vi "wavtest.vi"() -> ()   [LabVIEW 2016]
uses:
  <vilib>/Instr/_visa.llb/VISA Configure Serial Port (Instr).vi
  <vilib>/measure/maspectr.llb/FFT Spectrum (Mag-Phase) for 1 Chan.vi
  <vilib>/Waveform/WDTOps.llb/WDT Append Waveforms DBL.vi
  <vilib>/measure/NI_MAPro.lvlib
panel:
  out "VISA name":refnum<visa-resource-name>
  out "JSON string 2":string
  out "JSON string":string
  out "Para Cubo 2":dbl[][](array[numeric])
  out "# found 2":i32
  out "Janela 2":waveform(dbl)(graph)
  out "Amp 2":cluster{"f0":dbl, "df":dbl, "magnitude":dbl[]}(graph) caption="Amp"
  out "Raw Wave 2":waveform(dbl)(graph)
  in  "Record Button":bool caption="Gravar"
  in  "Close":bool
  out "Para Cubo":dbl[][](array[numeric])
  out "# found":i32
  in  "Tempo de Amostra do Som":dbl=0.01 min=0.05 max=1.0 step=0.01 format="%#_13g"
  out "Max iter":i32
  out "Ele/0,1s":dbl
  out "dt":dbl
  out "Duração Total":dbl
  out "size(s)":i32
  out "error out":errorcluster
  out "Janela":waveform(dbl)(graph)
  out "Amp":cluster{"f0":dbl, "df":dbl, "magnitude":dbl[]}(graph)
  in  "Play Button":bool
  out "Raw Wave":waveform(dbl)(graph)
  in  "Path to wav song":path caption="Escolher Arquivo"
  out "Menu 1":u32(colorbox)
  out "Ajustes":u32(colorbox)
  out "Back":u32(colorbox)
  # "Ajustes"
  # "PSI3214 -\nLaboratório de\nInstrumentação\nElétrica                 2016"
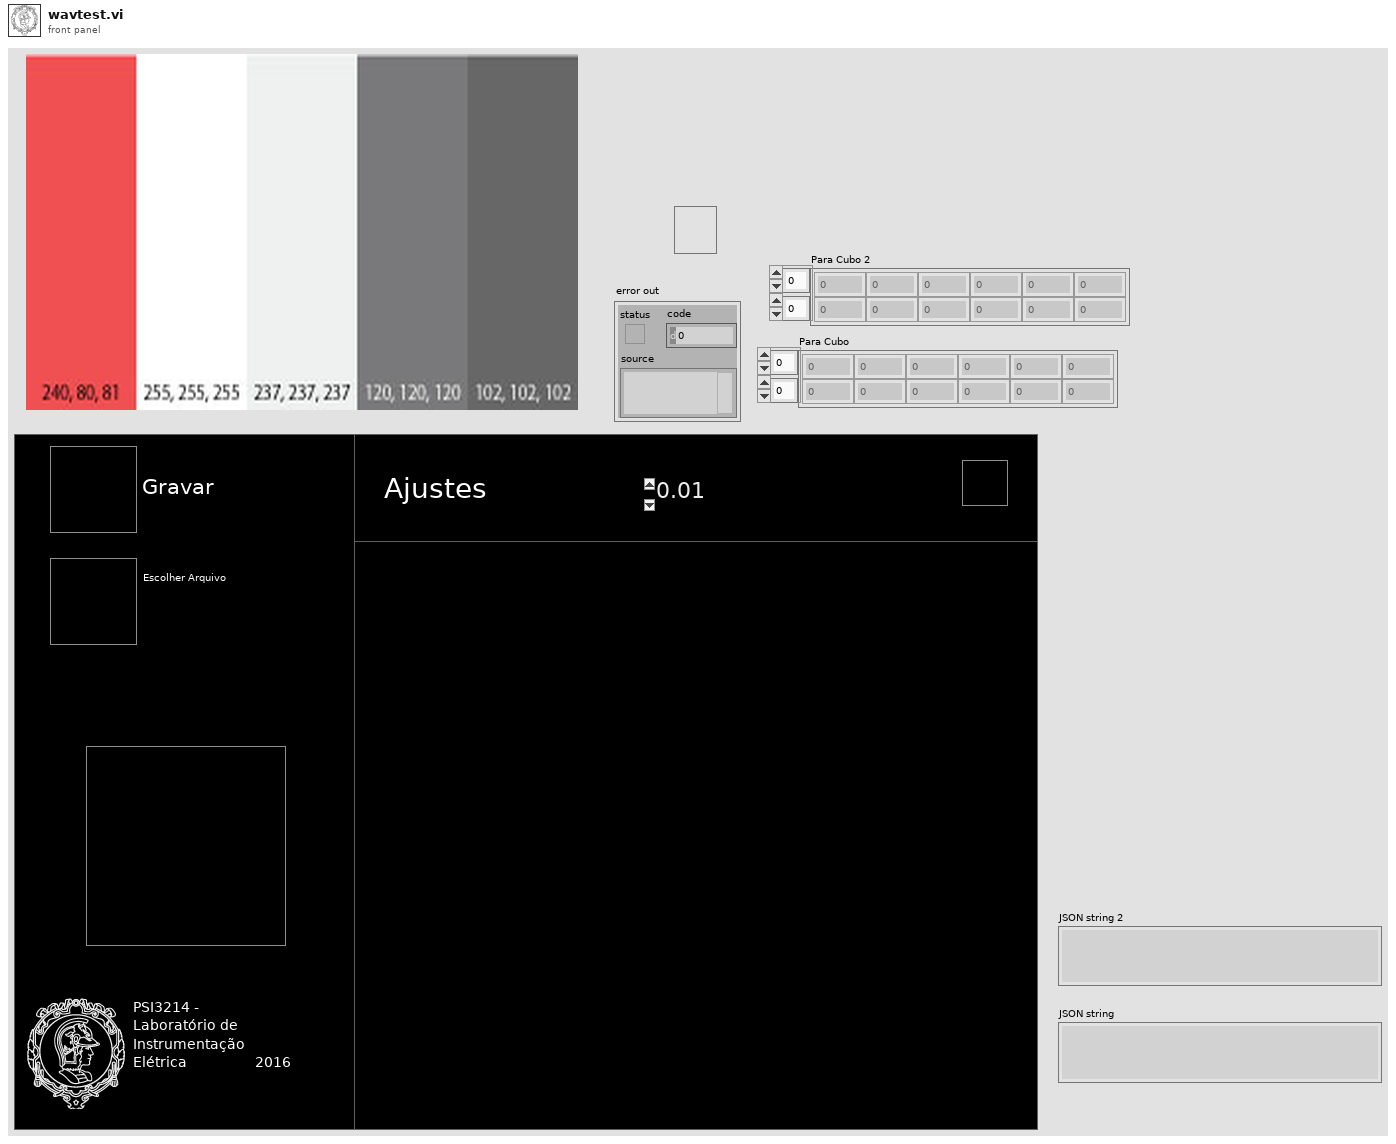
[diagram p1: front panel]
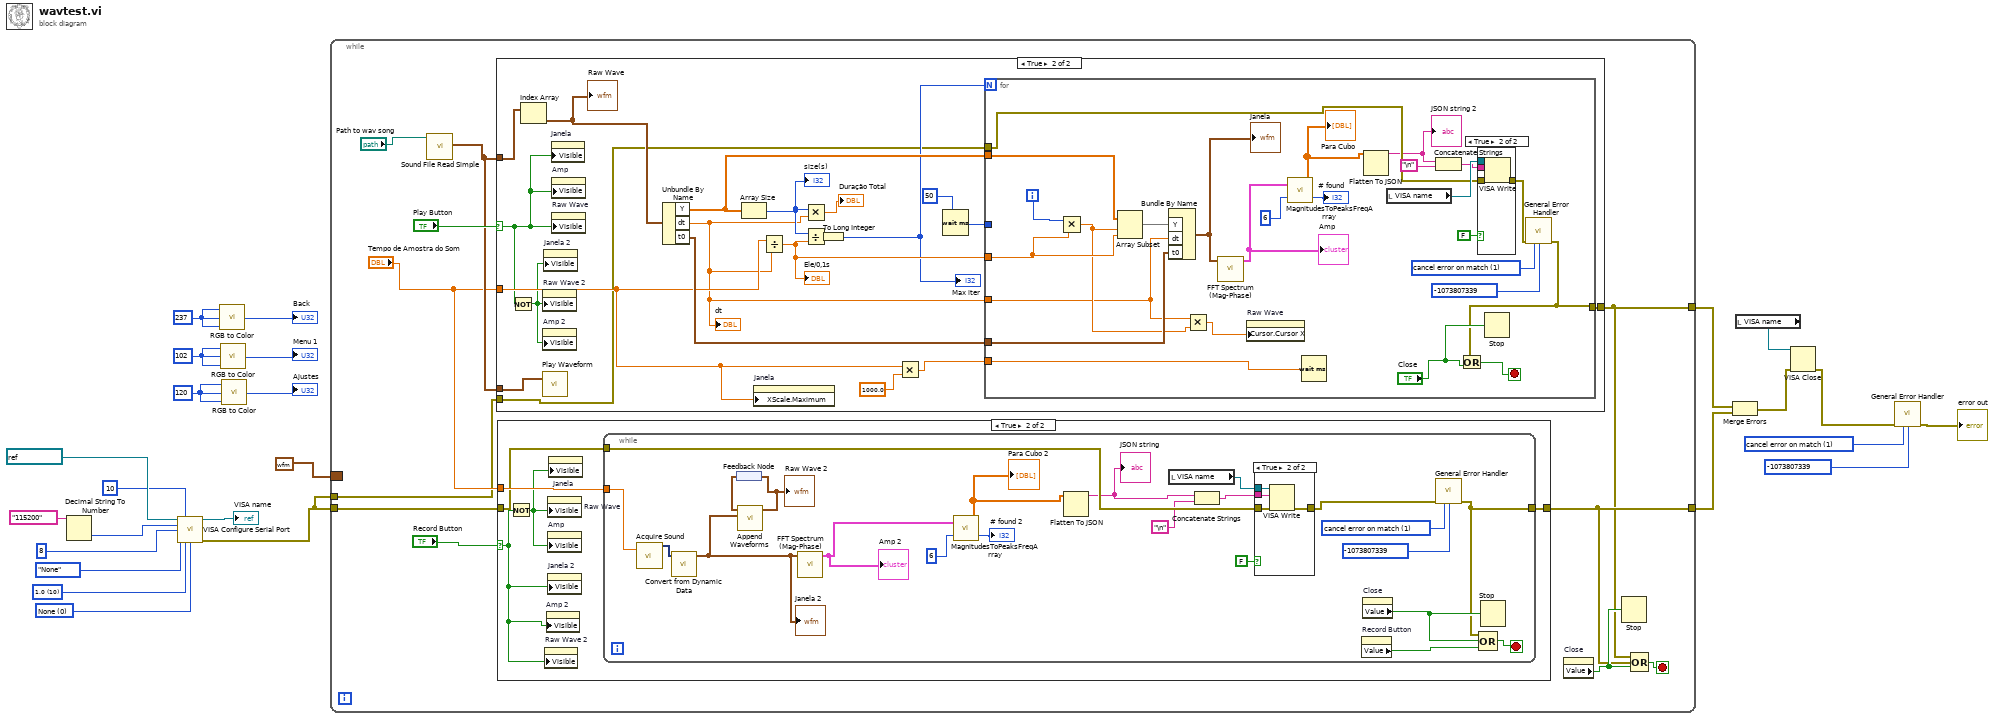
[diagram p0: block diagram]
diagram:
  w2 = 1 items=["no exception", "cancel error on match", "set error on match"] ("[exception action] (none:0)")
  w14 = u16 0 items=["None", "XON/XOFF", "RTS/CTS", "XON/XOFF & RTS/CTS", "DTR/DSR", "XON/XOFF & DTR/DSR"] ("flow control (0:none)")
  w15 = u16 10 items=["1.0"=10, "1.5"=15, "2.0"=20] ("stop bits (10: 1 bit)")
  w19 = u8 120 ("G")
  w20 = u8 102 ("G")
  w21 = u8 237 ("G")
  n1 = Decimal String To Number(string="115200" ("Baud Rate")) -> (number=w12:i32)  [unwired: 2 in, 1 out]
  n2 = call-poly "VISA Configure Serial Port"("VISA resource name"=refnum<visa-resource-name> "COM18" ("COM Port"), "timeout (10sec)"=u32 10, "baud rate (9600)"=w12, "data bits (8)"=u16 8, "parity (0:none)"=enum16{"None", "Odd", "Even", "Mark", "Space"}."None", "stop bits (10: 1 bit)"=w15, "flow control (0:none)"=w14) -> ("VISA resource name out"=→"VISA name":refnum<visa-resource-name>, "error out"=w4:errorcluster)  [unwired: 7 in]
  n3 = call <vilib>:"RGB to Color.vi"("B"=w21, "G"=w21, "R"=w21) -> ("Color"=→"Back":u32)
  n4 = call <vilib>:"RGB to Color.vi"("B"=w20, "G"=w20, "R"=w20) -> ("Color"=→"Menu 1":u32)
  n5 = call <vilib>:"RGB to Color.vi"("B"=w19, "G"=w19, "R"=w19) -> ("Color"=→"Ajustes":u32)
  n6 = while {
    border: waveform(dbl) {"t0"=timestamp(0 s since 1904-01-01), "dt"=1.0, "Y"=[]} ("waveform out") -> [_]
    tunnel: [w26] -> w7
    tunnel: [w27] -> w6
    tunnel: w4 -> [w31]
    tunnel: w4 -> [w30]
    stop <- w28 stop-if-true
    n7 = call <vilib>:"Sound File Read Simple.vi"("path"="Path to wav song") -> ("data"=w35:waveform(dbl)[])  [unwired: 7 in, 3 out]
    n8 = case shown="True" "Play Button" {
      selector: "Play Button" -> [_ w73]
      tunnel: w35 -> [_ w90]
      tunnel: "Tempo de Amostra do Som" -> [_ w79]
      tunnel: w35 -> [_ w75]
      tunnel: [w70 w72] -> w26
      tunnel: w30 -> [w70 w71]
      frame False {
      }
      frame True {
        n9 = Not(x=w73) -> (.not. x?=w74:bool)
        n10 = Index Array(array=w90) -> (element=w83:waveform(dbl))  [unwired: 1 in]
        "Raw Wave" <- w83
        n11 = call "Play Waveform"("Data"=w75) -> ()  [unwired: 18 in, 1 out]
        n12 = property on="Raw Wave 2" class="WFGraph (strict)"("Visible"=w74) -> ()  [unwired: 2 in, 2 out]
        n13 = property on="Amp 2" class="WFGraph (strict)"("Visible"=w74) -> ()  [unwired: 2 in, 2 out]
        n14 = property on="Janela 2" class="WFGraph (strict)"("Visible"=w74) -> ()  [unwired: 2 in, 2 out]
        n15 = property on="Janela" class="WFGraph (strict)"("Visible"=w73) -> ()  [unwired: 2 in, 2 out]
        n16 = property on="Amp" class="WFGraph (strict)"("Visible"=w73) -> ()  [unwired: 2 in, 2 out]
        n17 = property on="Raw Wave" class="WFGraph (strict)"("Visible"=w73) -> ()  [unwired: 2 in, 2 out]
        n18 = Unbundle By Name(w83) -> ("Y"=w86:dbl[], "dt"=w78:dbl, "t0"=w84:timestamp)
        "dt" <- w78
        n19 = Array Size(array=w86) -> (size(s)=w88:i32)
        "size(s)" <- w88
        n20 = property on="Janela" class="WFGraph (strict)"("XScale.Maximum"=w79) -> ()  [unwired: 2 in, 2 out]
        n21 = Divide(x=w79, y=w78) -> (x/y=w85:dbl)
        "Ele/0,1s" <- w85
        n22 = Multiply(x=w88, y=w78) -> (x*y=→"Duração Total":dbl)
        n23 = Divide(x=w88, y=w85) -> (x/y=w87:dbl)
        n24 = To Long Integer(number=w87) -> (32bit integer=w82:i32)
        "Max iter" <- w82
        n25 = Multiply(x=w79, y=1000.0) -> (x*y=w80:dbl)
        n26 = Wait (ms)(milliseconds to wait=u32 50) -> (millisecond timer value=w77:u32)
        n27 = for {
          N: w82 -> [_]
          tunnel: w86 -> [w116]
          tunnel: w85 -> [w114]
          tunnel: w84 -> [w113]
          tunnel: w80 -> [w111]
          tunnel: w78 -> [w106]
          tunnel: w77 -> [_]
          tunnel: [w93] -> w72
          tunnel: w71 -> [w99]
          i -> [w112]
          stop <- w100 stop-if-true
          w92 = 1 items=["no exception", "cancel error on match", "set error on match"] ("[exception action] (none:0)")
          n28 = Multiply(x=w112, y=w114) -> (x*y=w108:dbl)
          n29 = Array Subset(array=w116, index=w108, length=w114) -> (w115:dbl[])
          n30 = Bundle By Name("Y"=w115, "dt"=w106, "t0"=w113) -> (w110:waveform(dbl))  [unwired: 1 in]
          "Janela" <- w110
          n31 = Multiply(x=w106, y=w108) -> (x*y=w107:dbl)
          n32 = call-poly <vilib>:"FFT Spectrum (Mag-Phase).vi"("time signal"=w110) -> ("magnitude"=w109:cluster{"f0":dbl, "df":dbl, "magnitude":dbl[]})  [unwired: 6 in, 4 out]
          "Amp" <- w109
          n33 = property on="Raw Wave" class="WFGraph (strict)"("Cursor.Cursor X"=w107) -> ()  [unwired: 2 in, 2 out]
          n34 = call "MagnitudesToPeaksFreqArray.vi"("Size"=6, "magnitude"=w109) -> ("# found"=→"# found":i32, "Para Cubo"=w103:dbl[][])
          "Para Cubo" <- w103
          n35 = Wait (ms)(milliseconds to wait=w111) -> ()  [unwired: 1 out]
          n36 = Flatten To JSON(anything=w103) -> (JSON string=w98:string)  [unwired: 2 in, 1 out]
          "JSON string 2" <- w98
          n37 = local read "VISA name"() -> (w102:refnum<visa-resource-name>)
          n38 = Concatenate Strings(w98, "\n") -> (w96:string)
          n39 = case shown="True" FALSE {
            tunnel: w102 -> [_ w121]
            tunnel: [w117 w120] -> w94
            tunnel: w99 -> [w117 w119]
            tunnel: w96 -> [_ w118]
            frame False {
            }
            frame True {
              n40 = VISA Write(VISA resource name=w121, write buffer=w118, error in (no error)=w119) -> (error out=w120:errorcluster)  [unwired: 2 out]
            }
          }
          n41 = Stop(stop? (T)="Close") -> ()
          n42 = call <vilib>:"General Error Handler.vi"("error in (no error)"=w94, "[exception action] (none:0)"=w92, "[exception code]"=-1073807339) -> ("error out"=w93:errorcluster)  [unwired: 8 in, 4 out]
          n43 = Or(x=w93, y="Close") -> (x .or. y?=w100:bool)
        }
      }
    }
    n44 = case shown="True" "Record Button" {
      selector: "Record Button" -> [_ w41]
      tunnel: "Tempo de Amostra do Som" -> [_ w42]
      tunnel: [w37 w39] -> w27
      tunnel: w31 -> [w37 w38]
      frame False {
      }
      frame True {
        n45 = Not(x=w41) -> (.not. x?=w40:bool)
        n46 = property on="Raw Wave 2" class="WFGraph (strict)"("Visible"=w41) -> ()  [unwired: 2 in, 2 out]
        n47 = property on="Amp 2" class="WFGraph (strict)"("Visible"=w41) -> ()  [unwired: 2 in, 2 out]
        n48 = property on="Raw Wave" class="WFGraph (strict)"("Visible"=w40) -> ()  [unwired: 2 in, 2 out]
        n49 = property on="Amp" class="WFGraph (strict)"("Visible"=w40) -> ()  [unwired: 2 in, 2 out]
        n50 = property on="Janela 2" class="WFGraph (strict)"("Visible"=w41) -> ()  [unwired: 2 in, 2 out]
        n51 = property on="Janela" class="WFGraph (strict)"("Visible"=w40) -> ()  [unwired: 2 in, 2 out]
        n52 = while {
          tunnel: w42 -> [w64]
          tunnel: [w45] -> w39
          tunnel: w38 -> [w51]
          stop <- w52 stop-if-true
          w44 = 1 items=["no exception", "cancel error on match", "set error on match"] ("[exception action] (none:0)")
          n53 = call "Acquire Sound"("Duration (s)"=w64) -> ("Data"=w61:dynamicdata)  [unwired: 17 in, 1 out]
          n54 = call "Convert from Dynamic Data"("Dynamic Data Type"=w61) -> ("Waveform"=w58:waveform(dbl))  [unwired: 3 in]
          "Janela 2" <- w58
          n55 = feedback #1() -> (w59:waveform(dbl))
          n56 = call-poly <vilib>:"Append Waveforms.vi"("waveform B"=w58, "waveform A"=w59) -> ("waveform out"=w60:waveform(dbl))  [unwired: 8 in, 1 out]
          "Raw Wave 2" <- w60
          n57 = feedback-in #1(w60) -> ()
          n58 = call-poly <vilib>:"FFT Spectrum (Mag-Phase).vi"("time signal"=w58) -> ("magnitude"=w55:cluster{"f0":dbl, "df":dbl, "magnitude":dbl[]})  [unwired: 6 in, 4 out]
          "Amp 2" <- w55
          n59 = call "MagnitudesToPeaksFreqArray.vi"("Size"=6, "magnitude"=w55) -> ("# found"=→"# found 2":i32, "Para Cubo"=w54:dbl[][])
          "Para Cubo 2" <- w54
          n60 = Flatten To JSON(anything=w54) -> (JSON string=w50:string)  [unwired: 2 in, 1 out]
          "JSON string" <- w50
          n61 = local read "VISA name"() -> (w53:refnum<visa-resource-name>)
          n62 = Concatenate Strings(w50, "\n") -> (w49:string)
          n63 = case shown="True" FALSE {
            tunnel: w53 -> [_ w69]
            tunnel: [w65 w68] -> w46
            tunnel: w51 -> [w65 w67]
            tunnel: w49 -> [_ w66]
            frame False {
            }
            frame True {
              n64 = VISA Write(VISA resource name=w69, write buffer=w66, error in (no error)=w67) -> (error out=w68:errorcluster)  [unwired: 2 out]
            }
          }
          n65 = property on="Record Button" class="Bool (strict)"() -> ("Value"=w63:bool)  [unwired: 2 in, 2 out]
          n66 = property on="Close" class="Bool (strict)"() -> ("Value"=w62:bool)  [unwired: 2 in, 2 out]
          n67 = call <vilib>:"General Error Handler.vi"("error in (no error)"=w46, "[exception action] (none:0)"=w44, "[exception code]"=-1073807339) -> ("error out"=w45:errorcluster)  [unwired: 8 in, 4 out]
          n68 = Compound Arithmetic op=OR(w45, w62, w63) -> (w52:bool)
          n69 = Stop(stop? (T)=w62) -> ()
        }
      }
    }
    n70 = property on="Close" class="Bool (strict)"() -> ("Value"=w29:bool)  [unwired: 2 in, 2 out]
    n71 = Stop(stop? (T)=w29) -> ()
    n72 = Compound Arithmetic op=OR(w26, w27, w29) -> (w28:bool)
  }
  n73 = Merge Errors(w7, w6) -> (w5:errorcluster)
  n74 = local read "VISA name"() -> (w10:refnum<visa-resource-name>)
  n75 = VISA Close(VISA resource name=w10, error in (no error)=w5) -> (error out=w9:errorcluster)
  n76 = call <vilib>:"General Error Handler.vi"("error in (no error)"=w9, "[exception action] (none:0)"=w2, "[exception code]"=-1073807339) -> ("error out"=→"error out":errorcluster)  [unwired: 8 in, 4 out]
